vi "Worker CS Refs.vi"(11 "Work CS in":refnum<vi>) -> (0 "Tag In":refnum<vi>, 1 "Init In":refnum<vi>, 2 "Action In":refnum<vi>, 3 "Work CS":refnum<vi>, 4 "State In":refnum<vi>, 6 "State Out":refnum<vi>)   [LabVIEW 2020, in "FlexBlocks.lvlib"]
uses:
  FlexBlocks.lvlib
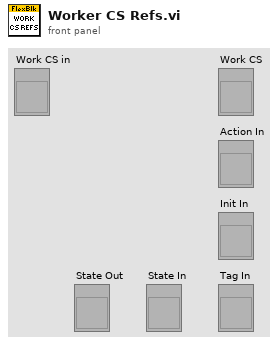
[diagram p1: front panel]
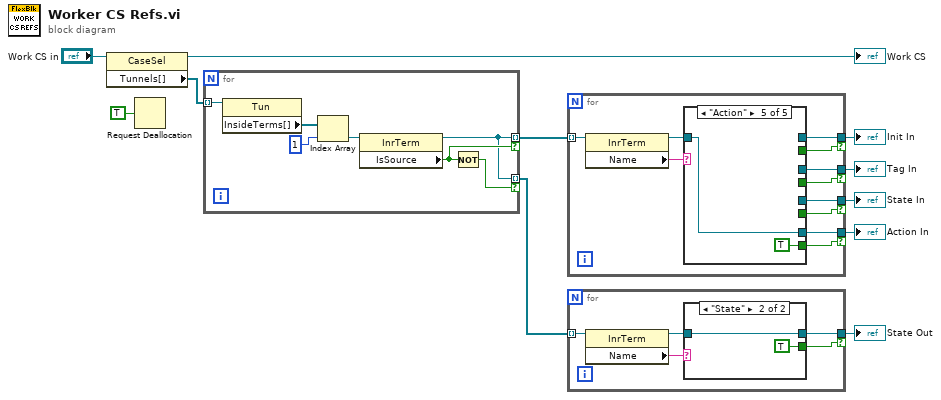
[diagram p0: block diagram]
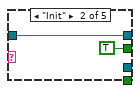
[diagram p4: hidden frame]
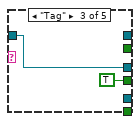
[diagram p5: hidden frame]
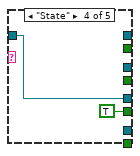
[diagram p6: hidden frame]
diagram:
  n1 = property class="CaseSel"(reference="Work CS in") -> (reference out=→"Work CS":refnum<vi>, "Tunnels[]"=w10:refnum<vi>[])  [unwired: 1 in, 1 out]
  n2 = Request Deallocation(TRUE ("flag")) -> ()
  n3 = for {
    tunnel: w10 -> [w18] mode=indexing
    tunnel: [w13] -> w9 mode=indexing if=w14
    tunnel: [w13] -> w7 mode=indexing if=w12
    n4 = property class="Tun"(reference=w18) -> ("InsideTerms[]"=w17:refnum<vi>[])  [unwired: 1 in, 2 out]
    n5 = Index Array(array=w17, index=1) -> (element=w15:refnum<vi>)
    n6 = property class="InrTerm"(reference=w15) -> (reference out=w13:refnum<vi>, "IsSource"=w14:bool)  [unwired: 1 in, 1 out]
    n7 = Not(x=w14) -> (.not. x?=w12:bool)
  }
  n8 = for {
    tunnel: w9 -> [w29] mode=indexing
    tunnel: [w26] -> w6 if=w25
    tunnel: [w23] -> w5 if=w24
    tunnel: [w19] -> w4 if=w20
    tunnel: [w22] -> w3 if=w21
    n9 = property class="InrTerm"(reference=w29) -> (reference out=w27:refnum<vi>, "Name"=w28:string)  [unwired: 1 in, 1 out]
    n10 = case shown="\"Action\"" w28 {
      tunnel: w27 -> [_ w31 w33 w35 w37]
      tunnel: [_ w31 _ _ _] -> w26
      tunnel: [_ TRUE _ _ _] -> w25
      tunnel: [_ _ w33 _ _] -> w23
      tunnel: [_ _ TRUE _ _] -> w24
      tunnel: [_ _ _ w35 _] -> w19
      tunnel: [_ _ _ TRUE _] -> w20
      tunnel: [_ _ _ _ w37] -> w22
      tunnel: [_ _ _ _ TRUE] -> w21
      frame Default {
      }
      frame "Init" {
      }
      frame "Tag" {
      }
      frame "State" {
      }
      frame "Action" {
      }
    }
  }
  "Init In" <- w6
  "Tag In" <- w5
  "State In" <- w4
  "Action In" <- w3
  n11 = for {
    tunnel: w7 -> [w42] mode=indexing
    tunnel: [w38] -> w2 if=w39
    n12 = property class="InrTerm"(reference=w42) -> (reference out=w40:refnum<vi>, "Name"=w41:string)  [unwired: 1 in, 1 out]
    n13 = case shown="\"State\"" w41 {
      tunnel: w40 -> [_ w44]
      tunnel: [_ w44] -> w38
      tunnel: [_ TRUE] -> w39
      frame Default {
      }
      frame "State" {
      }
    }
  }
  "State Out" <- w2
